vi "Set MessagePrefix.vi"(8 "error in (no error)":errorcluster, 10 "Message Prefix":string, 11 "PrefixQueue in":refnum<class "PrefixQueue.lvclass">) -> (0 "error out":errorcluster, 3 "PrefixQueue out":refnum<class "PrefixQueue.lvclass">)   [LabVIEW 2009, in "LapDog.Messaging.v2.PrefixQueue.lvlib" / "PrefixQueue.lvclass"]
doc: "Sets a text prefix that will be prepended to all message names. This can be useful when a message receiver needs to know the message sender's identity.\n\nThis method executes regardless of the error in state."
uses:
  PrefixQueue.lvclass
  PrefixQueue.lvclass/PrefixQueue.ctl
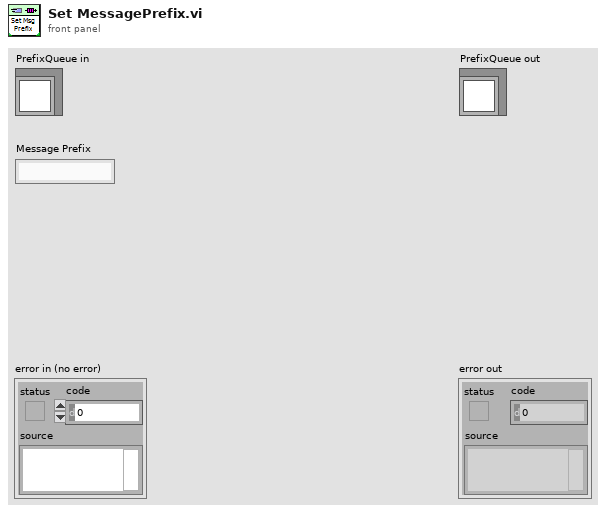
[diagram p1: front panel]
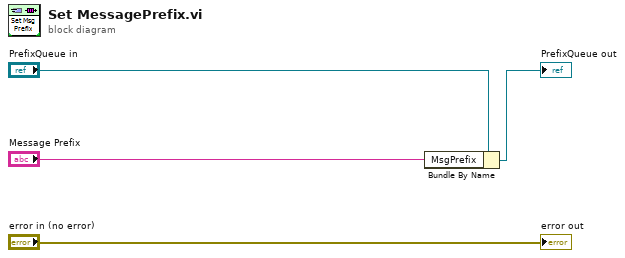
[diagram p0: block diagram]
diagram:
  n1 = Bundle By Name(cluster="PrefixQueue in", "MsgPrefix"="Message Prefix") -> (→"PrefixQueue out":refnum<class "PrefixQueue.lvclass">)
  "error out" <- "error in (no error)"
